vi "Modulator_USBSC.vi"(9 "Czas":dbl, 10 "Parametry_sygnalu_nosnego":T1, 11 "Sygnal_modulujacy":dbl[](array[numeric])) -> (3 "Sygnal_zmodulowany":dbl[](array[numeric]))   [LabVIEW 2020]
doc: "VI moduluje sygnal zmodulowany gornowstegowo"
uses:
  Kontrolki/Parametry_cosinusa.ctl
  <vilib>/Analysis/NI_AALPro.lvlib
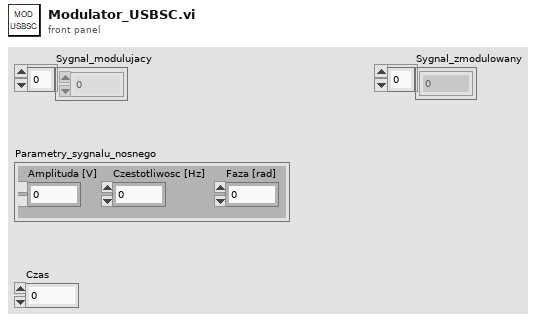
[diagram p1: front panel]
types:
  T1 = typedef "Parametry_cosinusa.ctl" = cluster{"Amplituda [V]":dbl, "Czestotliwosc [Hz] ":dbl, "Faza [rad]":dbl}
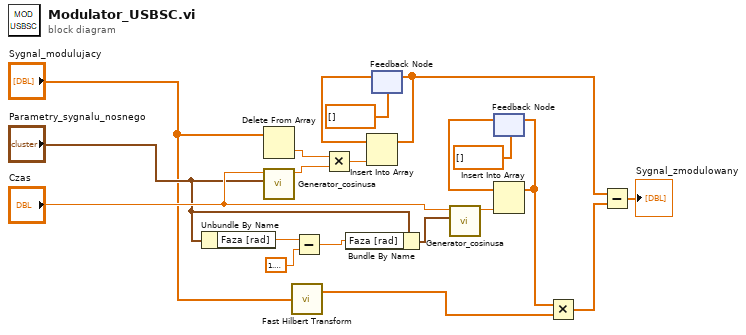
[diagram p0: block diagram]
diagram:
  n1 = Unbundle By Name("Parametry_sygnalu_nosnego") -> ("Faza [rad]"=w4:dbl)
  n2 = Delete From Array(array="Sygnal_modulujacy") -> (deleted portion=w9:dbl)  [unwired: 2 in, 1 out]
  n3 = call "Generator_cosinusa.vi"("Parametry_cosinusa"="Parametry_sygnalu_nosnego", "Czas"="Czas") -> ("A cos(2pift + phi)"=w8:dbl)  [unwired: 9 in]
  n4 = call <vilib>:"Fast Hilbert Transform.vi"("X"="Sygnal_modulujacy") -> ("Hilbert{X}"=w16:dbl[])  [unwired: 1 out]
  n5 = Subtract(x=w4, y=1.5707963267948966) -> (x-y=w5:dbl)
  n6 = Multiply(x=w9, y=w8) -> (x*y=w10:dbl)
  n7 = Bundle By Name(cluster="Parametry_sygnalu_nosnego", "Faza [rad]"=w5) -> (w7:T1)
  n8 = feedback #1(dbl[] []) -> (w12:dbl[])
  n9 = Insert Into Array(array=w12, new element=w10) -> (w19:dbl[])  [unwired: 1 in]
  n10 = feedback-in #1(w19) -> ()
  n11 = call "Generator_cosinusa.vi"("Parametry_cosinusa"=w7, "Czas"="Czas") -> ("A cos(2pift + phi)"=w13:dbl)  [unwired: 9 in]
  n12 = feedback #2(dbl[] []) -> (w15:dbl[])
  n13 = Insert Into Array(array=w15, new element=w13) -> (w17:dbl[])  [unwired: 1 in]
  n14 = feedback-in #2(w17) -> ()
  n15 = Multiply(x=w17, y=w16) -> (x*y=w18:dbl[])
  n16 = Subtract(x=w19, y=w18) -> (x-y=→"Sygnal_zmodulowany":dbl[])
